vi "Illini Hyperloop GUI v5.0.vi"() -> ()   [LabVIEW 2015]
uses:
  <vilib>/robotics/Controls/Attitude Indicator/Attitude Indicator.xctl
panel:
  out "True Position":dbl
  out "Voltage 2":dbl
  out "Voltage 1":dbl
  out "Ride Height Status":bool=TRUE
  out "Status Bits":u16 format="%b"
  out "Pressure Status":bool
  out "Temp Status":bool=TRUE
  out "Velocity Status":bool
  out "Position Status":bool
  out "Acceleration Status":bool
  out "Voltage Status":bool
  out "Current Status":bool
  out "Current 2":dbl
  out "Current 1":dbl
  in  "Pod State":u16(ring) items=["Pod Startup", "Safety Setup", "Safe Mode", "Functional Test", "Launch Ready", "Accel", "Coast", "Brake"]
  out "X2 Online":bool
  out "X1 Online":bool
  out "X2 Sen Stat":dbl
  out "X1 Sen Stat":dbl
  out "X2 State":dbl
  out "X1 State":dbl
  out "Position Chart":cluster{dbl, dbl, dbl}(graph)
  out "Brake Pressure":dbl
  out "RPM":dbl
  out "Accel 3":dbl
  out "Accel 2":dbl
  out "Accel 1":dbl
  out "True Accel":dbl
  out "True Velocity":dbl
  out "Pull Tab Disconnected":bool
  out "Currents":dbl(graph)
  out "Battery Voltages":cluster{dbl, dbl}(graph)
  out "Ride Height":cluster{u16, u16, u16}(graph)
  out "Y, Z Accel":cluster{u16, u16}(graph)
  out "Temp Chart":cluster{u16, u16, u16, u16, u16}(graph)
  out "Brake Pressure Chart":dbl(graph)
  out "Velocity chart":cluster{dbl, dbl}(graph)
  out "Optical Encoder Count":dbl
  out "Tape Count":dbl
  out "Acceleration Chart":cluster{dbl, dbl, dbl, dbl}(graph)
  in  "Send Command Button":bool
  in  "Command to Send":T1(ring)
  in  "Connection Status":enum16{"Disconnected", "Connected"}(ring)
  out "Attitude Indicator":cluster{"Roll":dbl, "Pitch":dbl}(xcontrol)
  in  "EMERGENCY BRAKE":bool
  in  "Functional Test Tab Control":enum32{"Network / File Info", "Program Control"}(tab)
  out "Client Closed":string="The client VI closed the connection."
  out "Most Recent Data":string
  in  "Connect to":string="192.168.137.100"
  in  "timeout ms":i32=1000
  in  "port":u16=8800
  in  "ms per loop":u32
  in  "bytes per write":i32=1000
  out "Base File Name":string
  in  "Stop Program":bool
  out "Producer Error Messages":errorcluster
  out "Consumer Error Messages":errorcluster
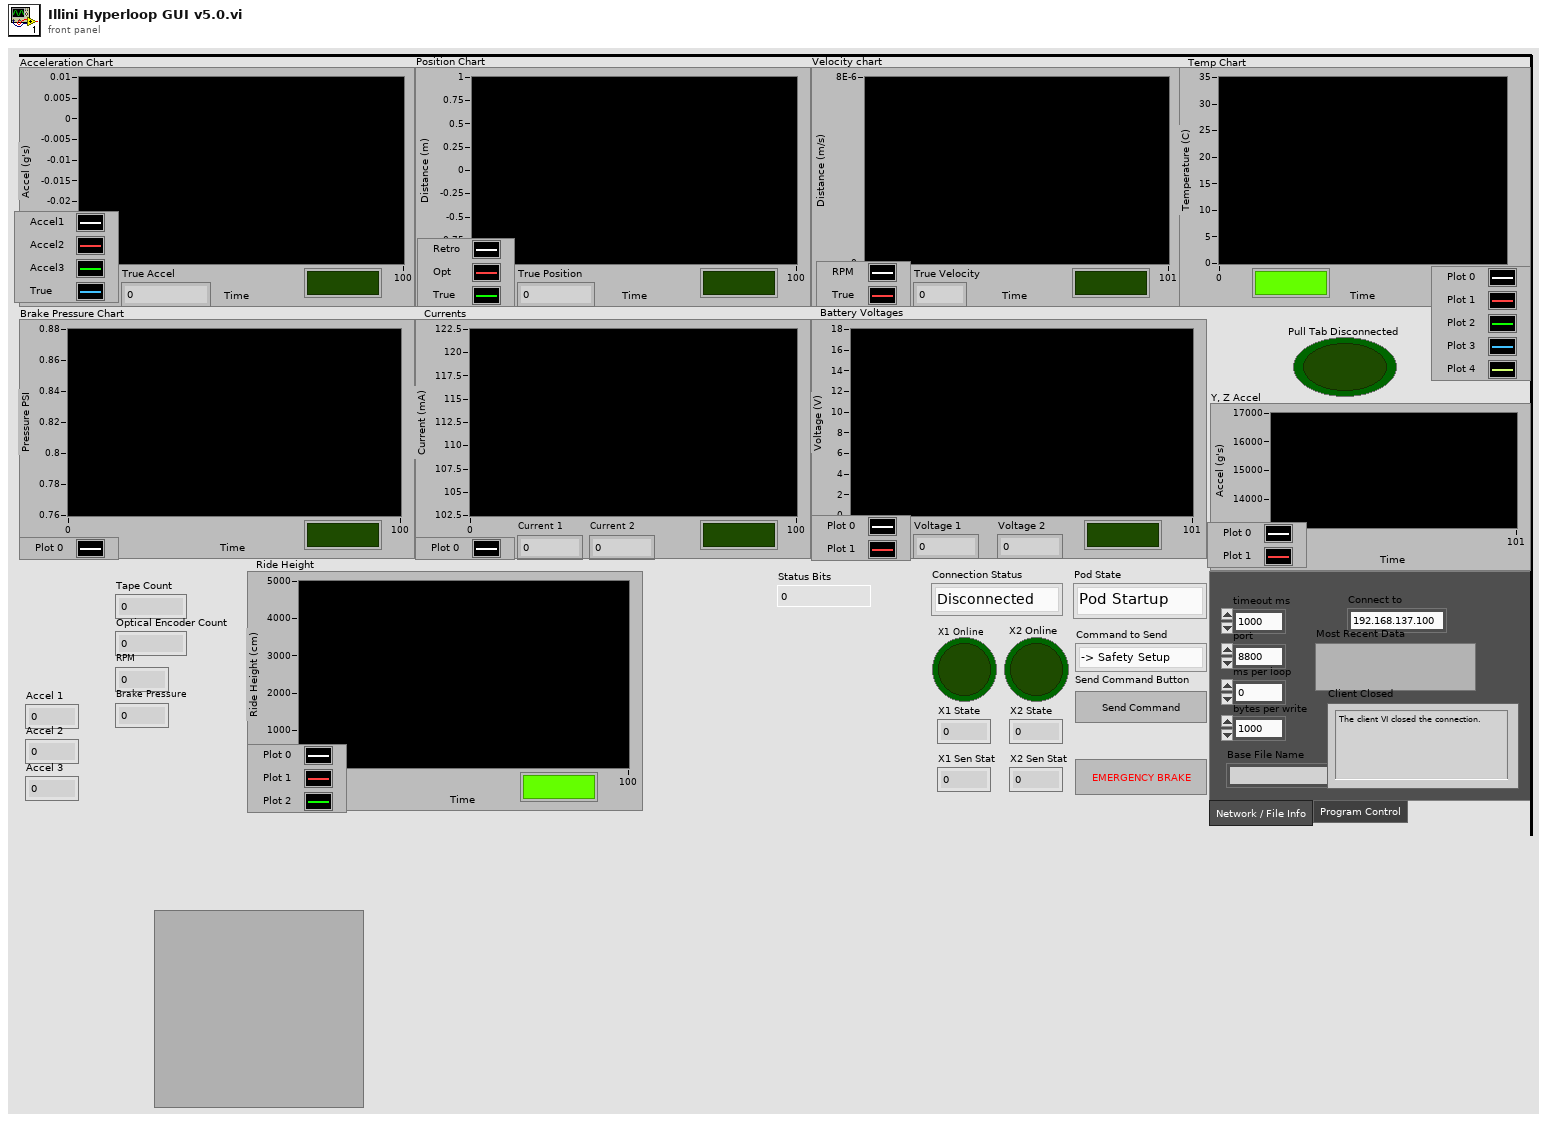
[diagram p1: front panel]
types:
  T1 = enum16{"-> Safety Setup", "-> Safe Mode", "-> Functional Test", "-> Ready to Launch", "-> Flight Brake", "EMERGENCY BRAKE", "Reset Sensors", "Calibrate Sensors", "Manual Brake ", "Manual Brake Reverse"}
  T2 = enum16{"Standard", "Buffered", "CRLF", "Immediate"}
  T3 = cluster{"Numeric 3":u16, "Numeric 3":u16, "Numeric 3":u16}
  T4 = cluster{"Tape Count":dbl, "Optical Encoder Count":dbl, "True Position":dbl}
  T5 = cluster{"Accel 1":dbl, "Accel 2":dbl, "Accel 3":dbl, "True Accel":dbl}
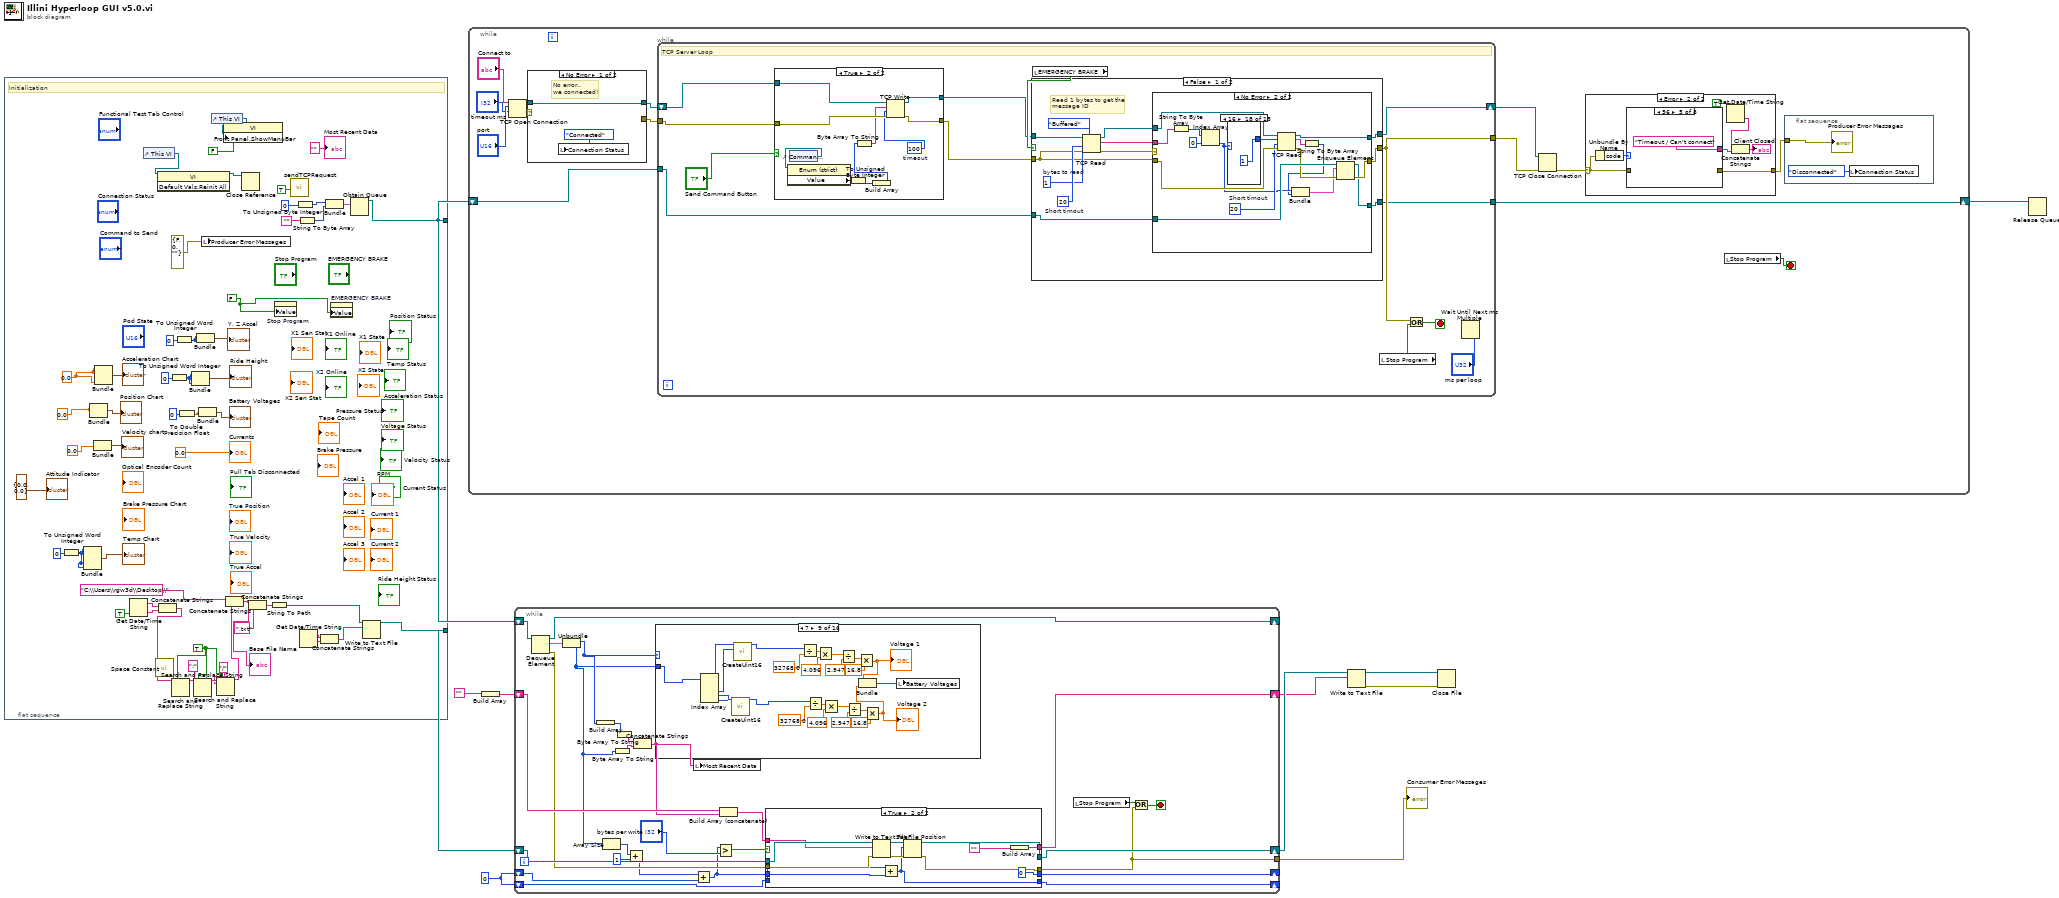
[diagram p0: block diagram]
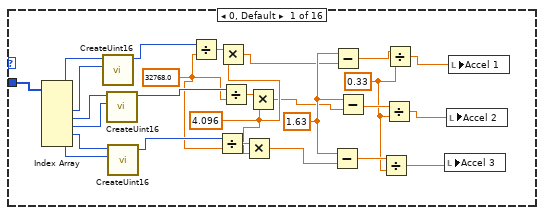
[diagram p2: hidden frame]
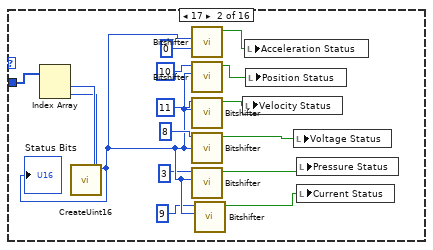
[diagram p3: hidden frame]
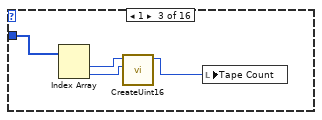
[diagram p4: hidden frame]
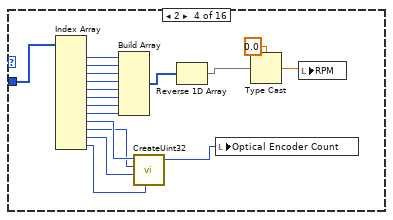
[diagram p5: hidden frame]
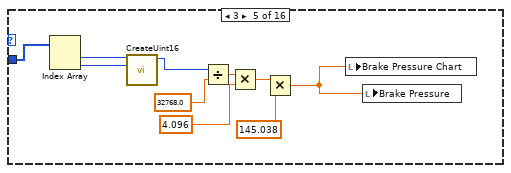
[diagram p6: hidden frame]
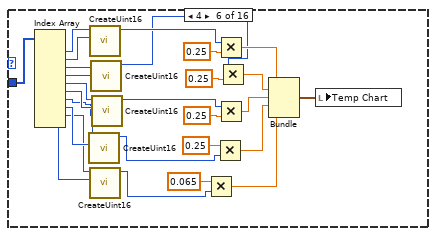
[diagram p7: hidden frame]
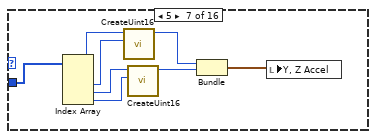
[diagram p8: hidden frame]
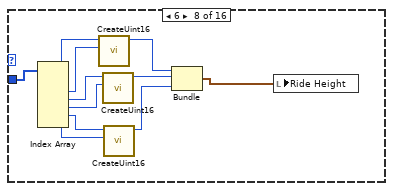
[diagram p9: hidden frame]
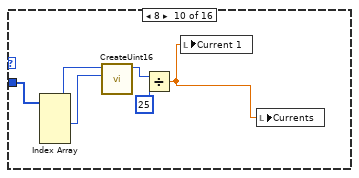
[diagram p10: hidden frame]
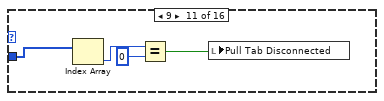
[diagram p11: hidden frame]
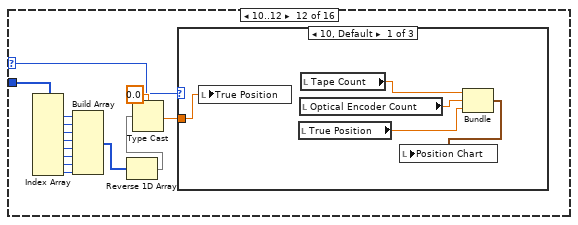
[diagram p12: hidden frame]
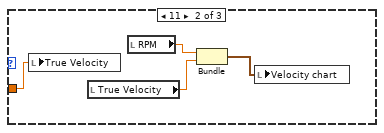
[diagram p13: hidden frame]
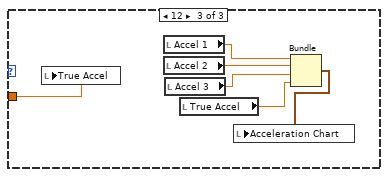
[diagram p14: hidden frame]
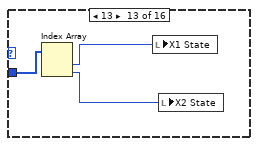
[diagram p15: hidden frame]
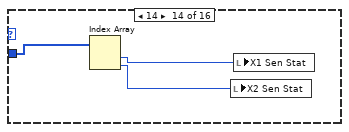
[diagram p16: hidden frame]
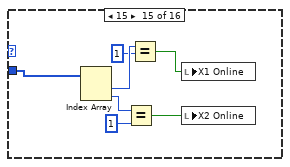
[diagram p17: hidden frame]
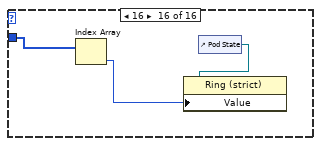
[diagram p18: hidden frame]
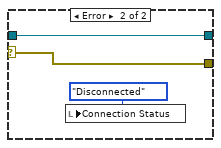
[diagram p20: hidden frame]
diagram:
  w2 = 0
  n1 = flat-sequence {
    tunnel: [w65] -> w11
    tunnel: [w52] -> w7
    frame #0 {
      w14 = 0.0
      w16 = 0.0
      w17 = 0.0
      w39 = TRUE ("want seconds? (F)")
      w62 = FALSE
      # "Initialization"
      n2 = To Unsigned Word Integer(number=0) -> (unsigned 16bit integer=w28:u16)
      n3 = Bundle(w28, w28, w28, w28, w28) -> (→"Temp Chart":cluster{u16, u16, u16, u16, u16})  [unwired: 1 in]
      n4 = Bundle(w14, w14, w14) -> (→"Position Chart":cluster{dbl, dbl, dbl})  [unwired: 1 in]
      n5 = Bundle(w16, w16) -> (→"Velocity chart":cluster{dbl, dbl})  [unwired: 1 in]
      n6 = Bundle(w17, w17, w17, w17) -> (→"Acceleration Chart":cluster{dbl, dbl, dbl, dbl})  [unwired: 1 in]
      n7 = Get Date/Time String(want seconds? (F)=TRUE) -> (date string=w50:string, time string=w49:string)  [unwired: 2 in]
      n8 = control-ref of="This VI"() -> (w57:refnum<vi>)
      n9 = call <vilib>:"Space Constant.vi"() -> ("String"=w51:string)
      n10 = invoke class="VI" method="Default Vals.Reinit All"(reference=w57) -> (reference out=w56:refnum<vi>)  [unwired: 2 in, 2 out]
      n11 = Concatenate Strings(w50, w49) -> (w48:string)
      n12 = To Unsigned Word Integer(number=0) -> (unsigned 16bit integer=w22:u16)
      n13 = Search and Replace String(replace all?=w39, input string=w48, search string=w51) -> (result string=w46:string)  [unwired: 5 in, 3 out]
      n14 = To Unsigned Word Integer(number=0) -> (unsigned 16bit integer=w25:u16)
      n15 = To Double Precision Float(number=0) -> (double precision float=w19:dbl)
      n16 = Bundle(w22, w22, w22) -> (→"Ride Height":cluster{u16, u16, u16})  [unwired: 1 in]
      n17 = Search and Replace String(replace all?=w39, input string=w46, search string=":" ("Functional Test 1 Data")) -> (result string=w42:string)  [unwired: 5 in, 3 out]
      n18 = Bundle(w25, w25) -> (→"Y, Z Accel":cluster{u16, u16})  [unwired: 1 in]
      n19 = Bundle(w19, w19) -> (→"Battery Voltages":cluster{dbl, dbl})  [unwired: 1 in]
      n20 = local write "Producer Error Messages"(errorcluster {"status"=FALSE, "code"=0, "source"=""} ("error constant")) -> ()
      n21 = control-ref of="This VI"() -> (w61:refnum<vi>)
      n22 = Search and Replace String(replace all?=w39, input string=w42, search string="/" ("Functional Test 1 Data")) -> (result string=w41:string)  [unwired: 5 in, 3 out]
      n23 = property class="VI"(reference=w61, "Front Panel.ShowMenuBar"=FALSE ("Front Panel Window:Show Menu Bar")) -> ()  [unwired: 1 in, 2 out]
      n24 = Concatenate Strings("C:\\Users\\rgw3d\\Desktop\\" ("Functional Test 1 Data"), w41) -> (w37:string)
      "Base File Name" <- w37
      n25 = Close Reference(reference=w56) -> ()  [unwired: 1 in, 1 out]
      n26 = Concatenate Strings(w37, ".txt" ("Functional Test 1 Data")) -> (w38:string)
      n27 = String To Path(string=w38) -> (path=w43:path)
      n28 = property on="Stop Program" class="Bool (strict)"("Value"=w62) -> ()  [unwired: 2 in, 2 out]
      n29 = call "sendTCPRequest.vi"("Force Reset"=TRUE) -> ()  [unwired: 9 in, 2 out]
      n30 = To Unsigned Byte Integer(number=0) -> (unsigned 8bit integer=w34:u8)
      n31 = String To Byte Array(string="") -> (unsigned byte array=w32:u8[])
      n32 = Get Date/Time String() -> (date string=w55:string, time string=w54:string)  [unwired: 3 in]
      n33 = Concatenate Strings(w55, w54) -> (w53:string)
      n34 = Bundle(w34, "unsigned byte array"=w32) -> (w31:cluster{u8, "unsigned byte array":u8[]})  [unwired: 1 in]
      n35 = property on="EMERGENCY BRAKE" class="Bool (strict)"("Value"=w62) -> ()  [unwired: 2 in, 2 out]
      n36 = Obtain Queue(element data type=w31) -> (queue out=w65:refnum<queue>)  [unwired: 4 in, 2 out]
      n37 = Write to Text File(file (use dialog)=w43, text=w53) -> (refnum out=w52:refnum<file>)  [unwired: 2 in, 2 out]
      "Attitude Indicator" <- cluster{"Roll":dbl, "Pitch":dbl} {"Roll"=0.0, "Pitch"=0.0} ("Attitude Indicator")
      "Most Recent Data" <- "" ("Data out")
      "Currents" <- 0.0
    }
  }
  n38 = while {
    shift-right: [w72] -> w1
    shift-left: w11 -> [w73]
    stop <- w69 stop-if-true
    n39 = TCP Open Connection(address="Connect to", remote port or service name="port", timeout ms (60000)="timeout ms") -> (connection ID=w74:refnum<k5>, error out=w75:errorcluster)  [unwired: 2 in]
    n40 = case shown="No Error" w75 {
      selector: w75 -> [_ w85]
      tunnel: w74 -> [w83 w86]
      tunnel: [w83 w86] -> w67
      tunnel: [_ w85] -> w66
      frame No Error {
        # "No error.. \nwe connected!"
        n41 = local write "Connection Status"(enum16{"Disconnected", "Connected"}."Connected" ("Connection Status")) -> ()
      }
      frame Error {
        n42 = local write "Connection Status"(enum16{"Disconnected", "Connected"}."Disconnected" ("Connection Status")) -> ()
      }
    }
    n43 = while {
      tunnel: w66 -> [w109]
      tunnel: [w114] -> w71
      tunnel: w73 -> [w108]
      tunnel: [w113] -> w72
      shift-right: [w112] -> w68
      shift-left: w67 -> [w110]
      stop <- w107 stop-if-true
      # "TCP Server Loop"
      n44 = case shown="True" "Send Command Button" {
        tunnel: w110 -> [w118 w128]
        tunnel: w109 -> [w117 w126]
        tunnel: [w117 w125] -> w105
        tunnel: [w118 w127] -> w106
        frame False {
        }
        frame True {
          w124 = 100  # timeout
          n45 = control-ref of="Command to Send"() -> (w123:refnum<vi>)
          n46 = property class="Enum (strict)"(reference=w123) -> ("Value"=w120:T1)  [unwired: 1 in, 2 out]
          n47 = To Unsigned Byte Integer(number=w120) -> (unsigned 8bit integer=w119:u8)
          n48 = Build Array(w119) -> (w122:u8[])
          n49 = Byte Array To String(unsigned byte array=w122) -> (string=w121:string)
          n50 = TCP Write(connection ID=w128, data in=w121, error in (no error)=w126, 9:w124) -> (connection ID out=w127:refnum<k5>, error out=w125:errorcluster)  [unwired: 1 out]
        }
      }
      n51 = local read "EMERGENCY BRAKE"() -> (w116:bool)
      n52 = case shown="False" w116 {
        tunnel: w105 -> [w137 w187]
        tunnel: w106 -> [w138 w186]
        tunnel: [w134 w185] -> w112
        tunnel: [w130 w184] -> w114
        tunnel: w108 -> [w132 w183]
        tunnel: [w131 w183] -> w113
        frame False {
          w139 = 1  # bytes to read
          w140 = 20  # Short timout
          # "Read 1 bytes to get the \nmessage ID"
          n53 = TCP Read(connection ID=w138, bytes to read=w139, error in (no error)=w137, 7:T2."Buffered" ("mode (standard)"), 9:w140) -> (connection ID out=w135:refnum<k5>, data out=w133:string, error out=w136:errorcluster)
          n54 = case shown="No Error" w136 {
            selector: w136 -> [w144 _]
            tunnel: w137 -> [w145 w156]
            tunnel: [w143 w163] -> w130
            tunnel: w135 -> [w142 w158]
            tunnel: [w142 w157] -> w134
            tunnel: w133 -> [_ w161]
            tunnel: w132 -> [w141 w164]
            tunnel: [w141 w162] -> w131
            frame Error {
              # "If the error code is 56 (no data available to read - which will happen when we are reading faster than the beaglebone can send data) Then parse out the error. \nIf the error code is not 56, then we have a problem"
              n55 = Unbundle By Name(w144) -> ("code"=w146:i32)
              n56 = case shown="56" w146 {
                tunnel: w144 -> [w147 _]
                tunnel: [w147 w148] -> w143
                tunnel: w145 -> [_ w148]
                frame Default {
                }
                frame 56 {
                }
              }
            }
            frame No Error {
              w154 = 20  # Short timout
              n57 = String To Byte Array(string=w161) -> (unsigned byte array=w159:u8[])
              n58 = Index Array(array=w159, index=0) -> (element=w152:u8)
              n59 = case shown="16" w152 {
                tunnel: [6 2 12 2 10 4 6 4 4 2 1 8 ("index") 8 ("index") 8 ("index") 2 ("index") 2 ("index") 2 ("index") 1 ("index")] -> w149
                frame 0, Default {
                }
                frame 1 {
                }
                frame 2 {
                }
                frame 3 {
                }
                frame 4 {
                }
                frame 5 {
                }
                frame 6 {
                }
                frame 7 {
                }
                frame 8 {
                }
                frame 17 {
                }
                frame 9 {
                }
                frame 10 {
                }
                frame 11 {
                }
                frame 12 {
                }
                frame 13 {
                }
                frame 14 {
                }
                frame 15 {
                }
                frame 16 {
                }
              }
              n60 = TCP Read(connection ID=w158, bytes to read=w149, error in (no error)=w156, 9:w154) -> (connection ID out=w157:refnum<k5>, data out=w151:string, error out=w155:errorcluster)  [unwired: 1 in]
              n61 = String To Byte Array(string=w151) -> (unsigned byte array=w150:u8[])
              n62 = Bundle(w152, "unsigned byte array"=w150) -> (w153:cluster{u8, "unsigned byte array":u8[]})  [unwired: 1 in]
              n63 = Enqueue Element(queue=w164, element=w153, error in (no error)=w155) -> (queue out=w162:refnum<queue>, error out=w163:errorcluster)  [unwired: 1 in, 1 out]
            }
          }
        }
        frame True {
          n64 = TCP Write(connection ID=w186, data in="OFF0000", error in (no error)=w187) -> (connection ID out=w185:refnum<k5>, error out=w184:errorcluster)  [unwired: 1 in, 1 out]
        }
      }
      n65 = local read "Stop Program"() -> (w115:bool)
      n66 = Or(x=w114, y=w115) -> (x .or. y?=w107:bool)
      n67 = Wait Until Next ms Multiple(millisecond multiple="ms per loop") -> ()  [unwired: 1 out]
    }
    n68 = TCP Close Connection(connection ID=w68, error in (no error)=w71) -> (error out=w79:errorcluster)  [unwired: 2 out]
    n69 = case shown="Error" w79 {
      selector: w79 -> [w87 w93]
      tunnel: [w87 w92] -> w78
      frame No Error {
      }
      frame Error {
        n70 = Unbundle By Name(w93) -> ("code"=w94:i32)
        n71 = case shown="56" w94 {
          tunnel: w93 -> [_ _ w98 _ _ _ _ _]
          tunnel: [_ _ w98 _ _ _ _ _] -> w92
          tunnel: ["The network is down, \nunreachable, or has been reset." "The specified network \naddress is currently in use." "Error" "The system caused the network \nconnection to be aborted." "Timeout / Can't connect" "Error 63. LabVIEW: The network connection \nwas refused by the server." "\tThe network connection\n is not yet established." "The network connection\n was closed by the peer."] -> w89
          frame 59 {
          }
          frame 60 {
          }
          frame Default {
          }
          frame 62 {
          }
          frame 56 {
          }
          frame 63 {
          }
          frame 64 {
          }
          frame 66 {
          }
        }
        n72 = Get Date/Time String(want seconds? (F)=TRUE) -> (time string=w90:string)  [unwired: 2 in, 1 out]
        n73 = Concatenate Strings(w90, w89) -> (→"Client Closed":string)
      }
    }
    n74 = local read "Stop Program"() -> (w69:bool)
    n75 = flat-sequence {
      tunnel: w78 -> [w81]
      frame #0 {
        n76 = local write "Connection Status"(enum16{"Disconnected", "Connected"}."Disconnected" ("Connection Status")) -> ()
        "Producer Error Messages" <- w81
      }
    }
  }
  n77 = Build Array("") -> (w8:string[])
  n78 = while {
    shift-right: [w216] -> _
    shift-left: w11 -> [w215]
    tunnel: [w205] -> w10
    shift-right: [w200] -> w3
    shift-left: w8 -> [w212]
    shift-right: [w210] -> w6
    shift-left: w7 -> [w211]
    shift-right: [w204] -> _
    shift-left: w2 -> [w208]
    shift-right: [w198] -> _
    shift-left: w2 -> [w199]
    stop <- w213 stop-if-true
    n79 = Dequeue Element(queue=w215) -> (queue out=w216:refnum<queue>, element=w209:cluster{u8, "unsigned byte array":u8[]}, error out=w207:errorcluster)  [unwired: 2 in, 1 out]
    n80 = Unbundle(w209) -> (w194:u8, "unsigned byte array"=w192:u8[])
    n81 = Build Array(w194) -> (w193:u8[])
    n82 = Array Size(array=w192) -> (size(s)=w197:i32)
    n83 = Byte Array To String(unsigned byte array=w192) -> (string=w191:string)
    n84 = Byte Array To String(unsigned byte array=w193) -> (string=w190:string)
    n85 = Add(x=w197, y=1) -> (x+y=w195:i32)
    n86 = Concatenate Strings(w190, w191) -> (w189:string)
    n87 = case shown="7" w194 {
      selector: w194 -> [_ _ _ _ _ _ _ _ _ _ _ w374 _ _ _ _]
      tunnel: w192 -> [w242 w258 w262 w280 w290 w315 w319 w327 w356 w365 w370 w375 w402 w405 w412 w415]
      frame 0, Default {
        w224 = 0.33 ("y")
        w220 = 1.63 ("y")
        w229 = 4.096 ("y")
        w228 = 32768.0
        n88 = Index Array(array=w242) -> (element #1=w241:u8, element #2=w240:u8, element #3=w239:u8, element #4=w238:u8, element #5=w237:u8, element #6=w236:u8)  [unwired: 6 in]
        n89 = call "CreateUint16.vi"("high"=w240, "low"=w241) -> ("Numeric 3"=w235:u16)  [unwired: 9 in]
        n90 = call "CreateUint16.vi"("high"=w238, "low"=w239) -> ("Numeric 3"=w230:u16)  [unwired: 9 in]
        n91 = call "CreateUint16.vi"("high"=w236, "low"=w237) -> ("Numeric 3"=w231:u16)  [unwired: 9 in]
        n92 = Divide(x=w235, y=w228) -> (x/y=w234:dbl)
        n93 = Divide(x=w231, y=w228) -> (x/y=w232:dbl)
        n94 = Multiply(x=w234, y=w229) -> (x*y=w219:dbl)
        n95 = Divide(x=w230, y=w228) -> (x/y=w233:dbl)
        n96 = Multiply(x=w232, y=w229) -> (x*y=w217:dbl)
        n97 = Multiply(x=w233, y=w229) -> (x*y=w218:dbl)
        n98 = Subtract(x=w220, y=w217) -> (x-y=w225:dbl)
        n99 = Subtract(x=w220, y=w219) -> (x-y=w227:dbl)
        n100 = Subtract(x=w220, y=w218) -> (x-y=w226:dbl)
        n101 = Divide(x=w225, y=w224) -> (x/y=w223:dbl)
        n102 = Divide(x=w226, y=w224) -> (x/y=w222:dbl)
        n103 = Divide(x=w227, y=w224) -> (x/y=w221:dbl)
        n104 = local write "Accel 3"(w223) -> ()
        n105 = local write "Accel 2"(w222) -> ()
        n106 = local write "Accel 1"(w221) -> ()
      }
      frame 17 {
        n107 = Index Array(array=w258) -> (element #1=w257:u8, element #2=w256:u8)  [unwired: 2 in]
        n108 = call "CreateUint16.vi"("high"=w256, "low"=w257) -> ("Numeric 3"=w245:u16)  [unwired: 9 in]
        "Status Bits" <- w245
        n109 = call "Bitshifter.vi"("Bits"=w245, "Type"=0) -> ("Output"=w254:bool)  [unwired: 9 in]
        n110 = call "Bitshifter.vi"("Bits"=w245, "Type"=10) -> ("Output"=w253:bool)  [unwired: 9 in]
        n111 = call "Bitshifter.vi"("Bits"=w245, "Type"=11) -> ("Output"=w250:bool)  [unwired: 9 in]
        n112 = call "Bitshifter.vi"("Bits"=w245, "Type"=8) -> ("Output"=w248:bool)  [unwired: 9 in]
        n113 = call "Bitshifter.vi"("Bits"=w245, "Type"=3) -> ("Output"=w247:bool)  [unwired: 9 in]
        n114 = call "Bitshifter.vi"("Bits"=w245, "Type"=9) -> ("Output"=w246:bool)  [unwired: 9 in]
        n115 = local write "Velocity Status"(w250) -> ()
        n116 = local write "Acceleration Status"(w254) -> ()
        n117 = local write "Position Status"(w253) -> ()
        n118 = local write "Voltage Status"(w248) -> ()
        n119 = local write "Pressure Status"(w247) -> ()
        n120 = local write "Current Status"(w246) -> ()
      }
      frame 1 {
        n121 = Index Array(array=w262) -> (element #1=w261:u8, element #2=w260:u8)  [unwired: 2 in]
        n122 = call "CreateUint16.vi"("high"=w260, "low"=w261) -> ("Numeric 3"=w259:u16)  [unwired: 9 in]
        n123 = local write "Tape Count"(w259) -> ()
      }
      frame 2 {
        n124 = Index Array(array=w280) -> (element #1=w273:u8, element #2=w272:u8, element #3=w271:u8, element #4=w270:u8, element #5=w269:u8, element #6=w268:u8, element #7=w267:u8, element #8=w266:u8, element #9=w279:u8, element #10=w278:u8, element #11=w277:u8, element #12=w276:u8)  [unwired: 12 in]
        n125 = Build Array(w273, w272, w271, w270, w269, w268, w267, w266) -> (w264:u8[])
        n126 = call "CreateUint32.vi"("Numeric in"=w276, "Numeric 3"=w277, "Numeric 4"=w278, "Numeric 5"=w279) -> ("Numeric out"=w275:u32)  [unwired: 7 in]
        n127 = Reverse 1D Array(array=w264) -> (reversed array=w263:u8[])
        n128 = local write "Optical Encoder Count"(w275) -> ()
        n129 = Type Cast(type=0.0, x=w263) -> (*(type *) &x=w265:dbl)
        n130 = local write "RPM"(w265) -> ()
      }
      frame 3 {
        n131 = Index Array(array=w290) -> (element #1=w289:u8, element #2=w288:u8)  [unwired: 2 in]
        n132 = call "CreateUint16.vi"("high"=w288, "low"=w289) -> ("Numeric 3"=w285:u16)  [unwired: 9 in]
        n133 = Divide(x=w285, y=32768.0) -> (x/y=w287:dbl)
        n134 = Multiply(x=w287, y=4.096) -> (x*y=w283:dbl)
        n135 = Multiply(x=w283, y=145.038) -> (x*y=w281:dbl)
        n136 = local write "Brake Pressure Chart"(w281) -> ()
        n137 = local write "Brake Pressure"(w281) -> ()
      }
      frame 4 {
        n138 = Index Array(array=w315) -> (element #1=w317:u8, element #2=w316:u8, element #3=w314:u8, element #4=w313:u8, element #5=w312:u8, element #6=w311:u8, element #7=w310:u8, element #8=w309:u8, element #9=w308:u8, element #10=w307:u8)  [unwired: 10 in]
        n139 = call "CreateUint16.vi"("high"=w309, "low"=w310) -> ("Numeric 3"=w296:u16)  [unwired: 9 in]
        n140 = call "CreateUint16.vi"("high"=w316, "low"=w317) -> ("Numeric 3"=w304:u16)  [unwired: 9 in]
        n141 = call "CreateUint16.vi"("high"=w307, "low"=w308) -> ("Numeric 3"=w294:u16)  [unwired: 9 in]
        n142 = call "CreateUint16.vi"("high"=w313, "low"=w314) -> ("Numeric 3"=w302:u16)  [unwired: 9 in]
        n143 = call "CreateUint16.vi"("high"=w311, "low"=w312) -> ("Numeric 3"=w297:u16)  [unwired: 9 in]
        n144 = Multiply(x=0.065 ("y"), y=w294) -> (x*y=w291:dbl)
        n145 = Multiply(x=0.25 ("y"), y=w296) -> (x*y=w292:dbl)
        n146 = Multiply(x=w304, y=0.25) -> (x*y=w303:dbl)
        n147 = Multiply(x=w297, y=0.25) -> (x*y=w293:dbl)
        n148 = Multiply(x=w302, y=0.25) -> (x*y=w300:dbl)
        n149 = Bundle(w303, w300, w293, w292, w291) -> (w306:cluster{dbl, dbl, dbl, dbl, dbl})  [unwired: 1 in]
        n150 = local write "Temp Chart"(w306) -> ()
      }
      frame 5 {
        n151 = Index Array(array=w319) -> (element #1=w324:u8, element #2=w323:u8, element #3=w322:u8, element #4=w321:u8)  [unwired: 4 in]
        n152 = call "CreateUint16.vi"("high"=w323, "low"=w324) -> ("Numeric 3"=w325:u16)  [unwired: 9 in]
        n153 = call "CreateUint16.vi"("high"=w321, "low"=w322) -> ("Numeric 3"=w320:u16)  [unwired: 9 in]
        n154 = Bundle("Numeric 3"=w325, "Numeric 3"=w320) -> (w318:cluster{"Numeric 3":u16, "Numeric 3":u16})  [unwired: 1 in]
        n155 = local write "Y, Z Accel"(w318) -> ()
      }
      frame 6 {
        n156 = Index Array(array=w327) -> (element #1=w335:u8, element #2=w334:u8, element #3=w333:u8, element #4=w332:u8, element #5=w331:u8, element #6=w330:u8)  [unwired: 6 in]
        n157 = call "CreateUint16.vi"("high"=w334, "low"=w335) -> ("Numeric 3"=w336:u16)  [unwired: 9 in]
        n158 = call "CreateUint16.vi"("high"=w332, "low"=w333) -> ("Numeric 3"=w329:u16)  [unwired: 9 in]
        n159 = call "CreateUint16.vi"("high"=w330, "low"=w331) -> ("Numeric 3"=w328:u16)  [unwired: 9 in]
        n160 = Bundle("Numeric 3"=w336, "Numeric 3"=w329, "Numeric 3"=w328) -> (w326:T3)  [unwired: 1 in]
        n161 = local write "Ride Height"(w326) -> ()
      }
      frame 7 {
        n162 = Index Array(array=w356) -> (element #1=w360:u8, element #2=w359:u8, element #3=w358:u8, element #4=w357:u8)  [unwired: 4 in]
        n163 = call "CreateUint16.vi"("high"=w357, "low"=w358) -> ("Numeric 3"=w339:u16)  [unwired: 9 in]
        n164 = call "CreateUint16.vi"("high"=w359, "low"=w360) -> ("Numeric 3"=w353:u16)  [unwired: 9 in]
        n165 = Divide(x=w353, y=32768.0) -> (x/y=w354:dbl)
        n166 = Divide(x=w339, y=32768.0) -> (x/y=w346:dbl)
        n167 = Multiply(x=w354, y=4.096) -> (x*y=w350:dbl)
        n168 = Multiply(x=w346, y=4.096) -> (x*y=w343:dbl)
        n169 = Divide(x=w350, y=2.947) -> (x/y=w348:dbl)
        n170 = Divide(x=w343, y=2.947) -> (x/y=w341:dbl)
        n171 = Multiply(x=w348, y=16.8) -> (x*y=w338:dbl)
        "Voltage 1" <- w338
        n172 = Multiply(x=w341, y=16.8) -> (x*y=w337:dbl)
        "Voltage 2" <- w337
        n173 = Bundle(w338, w337) -> (w355:cluster{dbl, dbl})  [unwired: 1 in]
        n174 = local write "Battery Voltages"(w355) -> ()
      }
      frame 8 {
        n175 = Index Array(array=w365) -> (element #1=w364:u8, element #2=w366:u8)  [unwired: 4 in, 2 out]
        n176 = call "CreateUint16.vi"("high"=w366, "low"=w364) -> ("Numeric 3"=w363:u16)  [unwired: 9 in]
        n177 = Divide(x=w363, y=u16 25) -> (x/y=w361:dbl)
        n178 = local write "Current 1"(w361) -> ()
        n179 = local write "Currents"(w361) -> ()
      }
      frame 9 {
        n180 = Index Array(array=w370) -> (element=w369:u8)  [unwired: 1 in]
        n181 = Equal?(x=w369, y=u8 0) -> (x = y?=w367:bool)
        n182 = local write "Pull Tab Disconnected"(w367) -> ()
      }
      frame 10..12 {
        n183 = Index Array(array=w375) -> (element #1=w383:u8, element #2=w382:u8, element #3=w381:u8, element #4=w380:u8, element #5=w379:u8, element #6=w378:u8, element #7=w377:u8, element #8=w376:u8)  [unwired: 8 in]
        n184 = Build Array(w383, w382, w381, w380, w379, w378, w377, w376) -> (w372:u8[])
        n185 = Reverse 1D Array(array=w372) -> (reversed array=w371:u8[])
        n186 = Type Cast(type=0.0, x=w371) -> (*(type *) &x=w373:dbl)
        n187 = case shown="10, Default" w374 {
          tunnel: w373 -> [w389 w393 w399]
          frame 10, Default {
            n188 = local write "True Position"(w389) -> ()
            n189 = local read "True Position"() -> (w386:dbl)
            n190 = local read "Optical Encoder Count"() -> (w387:dbl)
            n191 = local read "Tape Count"() -> (w388:dbl)
            n192 = Bundle("Tape Count"=w388, "Optical Encoder Count"=w387, "True Position"=w386) -> (w385:T4)  [unwired: 1 in]
            n193 = local write "Position Chart"(w385) -> ()
          }
          frame 11 {
            n194 = local write "True Velocity"(w393) -> ()
            n195 = local read "True Velocity"() -> (w390:dbl)
            n196 = local read "RPM"() -> (w391:dbl)
            n197 = Bundle("RPM"=w391, "True Velocity"=w390) -> (w392:cluster{"RPM":dbl, "True Velocity":dbl})  [unwired: 1 in]
            n198 = local write "Velocity chart"(w392) -> ()
          }
          frame 12 {
            n199 = local write "True Accel"(w399) -> ()
            n200 = local read "Accel 1"() -> (w398:dbl)
            n201 = local read "Accel 2"() -> (w397:dbl)
            n202 = local read "Accel 3"() -> (w396:dbl)
            n203 = local read "True Accel"() -> (w395:dbl)
            n204 = Bundle("Accel 1"=w398, "Accel 2"=w397, "Accel 3"=w396, "True Accel"=w395) -> (w394:T5)  [unwired: 1 in]
            n205 = local write "Acceleration Chart"(w394) -> ()
          }
        }
      }
      frame 13 {
        n206 = Index Array(array=w402) -> (element #1=w401:u8, element #2=w400:u8)  [unwired: 2 in]
        n207 = local write "X1 State"(w401) -> ()
        n208 = local write "X2 State"(w400) -> ()
      }
      frame 14 {
        n209 = Index Array(array=w405) -> (element #1=w404:u8, element #2=w403:u8)  [unwired: 2 in]
        n210 = local write "X2 Sen Stat"(w403) -> ()
        n211 = local write "X1 Sen Stat"(w404) -> ()
      }
      frame 15 {
        n212 = Index Array(array=w412) -> (element #1=w411:u8, element #2=w409:u8)  [unwired: 2 in]
        n213 = Equal?(x=w409, y=u8 1) -> (x = y?=w407:bool)
        n214 = Equal?(x=w411, y=u8 1) -> (x = y?=w406:bool)
        n215 = local write "X1 Online"(w406) -> ()
        n216 = local write "X2 Online"(w407) -> ()
      }
      frame 16 {
        n217 = Index Array(array=w415) -> (element=w413:u8)  [unwired: 1 in]
        n218 = control-ref of="Pod State"() -> (w414:refnum<vi>)
        n219 = property class="Ring (strict)"(reference=w414, "Value"=w413) -> ()  [unwired: 1 in, 2 out]
      }
    }
    n220 = local write "Most Recent Data"(w189) -> ()
    n221 = Add(x=w195, y=w208) -> (x+y=w201:i32)
    n222 = Greater?(x=w201, y="bytes per write") -> (0:w206:bool)
    n223 = Build Array (concatenate)(w212, w189) -> (w202:string[])
    n224 = case shown="True" w206 {
      tunnel: w202 -> [w417 w424]
      tunnel: w211 -> [w420 w433]
      tunnel: [w420 w427] -> w210
      tunnel: w201 -> [w419 w422]
      tunnel: [w418 w430] -> w205
      tunnel: w207 -> [w418 w429]
      tunnel: [w419 0] -> w204
      tunnel: [w417 w425] -> w200
      tunnel: w199 -> [w416 w423]
      tunnel: [w416 w421] -> w198
      frame False {
      }
      frame True {
        n225 = Write to Text File(file (use dialog)=w433, text=w424, error in=w429) -> (refnum out=w432:refnum<file>, error out=w431:errorcluster)  [unwired: 1 in, 1 out]
        n226 = Add(x=w423, y=w422) -> (x+y=w421:i32)
        n227 = Set File Position(offset (in bytes) (0)=w421, refnum=w432, error in=w431) -> (refnum out=w427:refnum<file>, error out=w430:errorcluster)  [unwired: 1 in]
        n228 = Build Array("") -> (w425:string[])
      }
    }
    n229 = local read "Stop Program"() -> (w214:bool)
    n230 = Or(x=w214, y=w205) -> (x .or. y?=w213:bool)
  }
  "Consumer Error Messages" <- w10
  n231 = Write to Text File(file (use dialog)=w6, text=w3) -> (refnum out=w4:refnum<file>, error out=w5:errorcluster)  [unwired: 2 in, 1 out]
  n232 = Close File(refnum=w4, error in=w5) -> ()  [unwired: 2 out]
  n233 = Release Queue(queue=w1) -> ()  [unwired: 2 in, 3 out]
